vi "Configure.vi"(8 "error in (no error)":errorcluster, 11 "Autofocus in":refnum<class "Autofocus.lvclass">) -> (0 "error out":errorcluster, 2 "cancelled?":bool, 3 "Autofocus out":refnum<class "Autofocus.lvclass">)   [LabVIEW 2012, in "Autofocus.lvclass"]
doc: "The configure method configures the details for the RabbitMQ connection, the observers and the mapping script.\n\nIn the derived class, make a call to the parent for setting these parameters."
uses:
  Autofocus.lvclass
  number of subregions.ctl
  <vilib>/Utility/miscctls.llb/LVPointTypeDef.ctl
  Autofocus.lvclass/Autofocus.ctl
  <vilib>/Distrio/Murmex/Murmex/Murmex.lvclass
panel:
  in  "button::ok":bool
  in  "button::configure murmex":bool
  in  "button::cancel":bool
  in  "Tab Control":enum32{"Component IDs", "Search parameters"}(tab)
  in  "AOTF component name":string
  in  "Camera component name":string
  in  "Stages component name":string
  in  "Epsilon (HC)":dbl
  in  "Epsilon (GS)":dbl
  in  "Number of subregions":T1 items=["4"=4, "5"=5]
  # "RabbitMQ parameters"
  # "Window position"
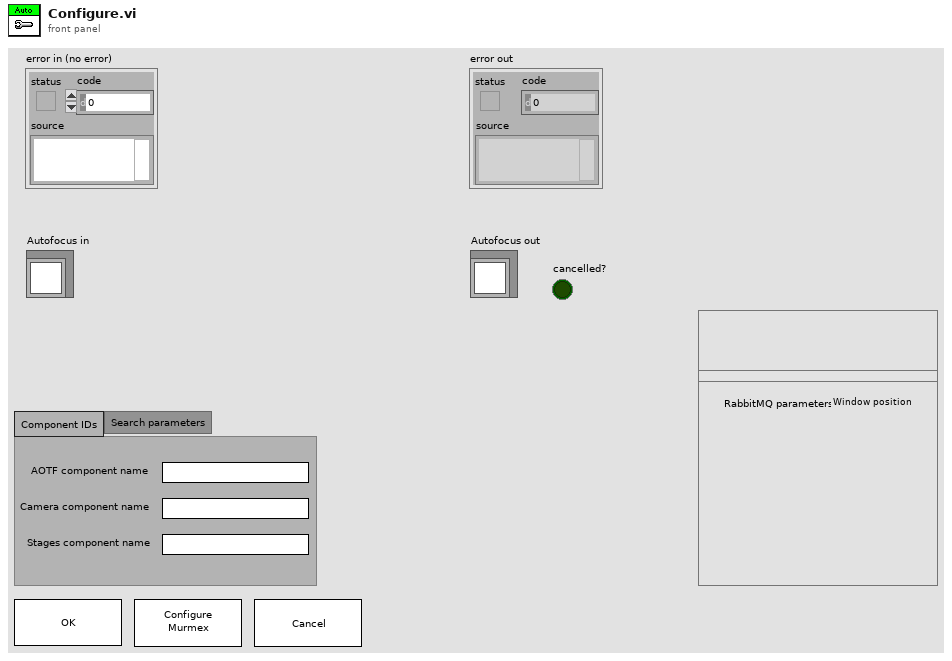
[diagram p1: front panel]
types:
  T1 = typedef "Autofocus.lvclass/number of subregions.ctl" = i32
  T2 = typedef "LVPointTypeDef.ctl" = cluster{"Horizontal":i16, "Vertical":i16}
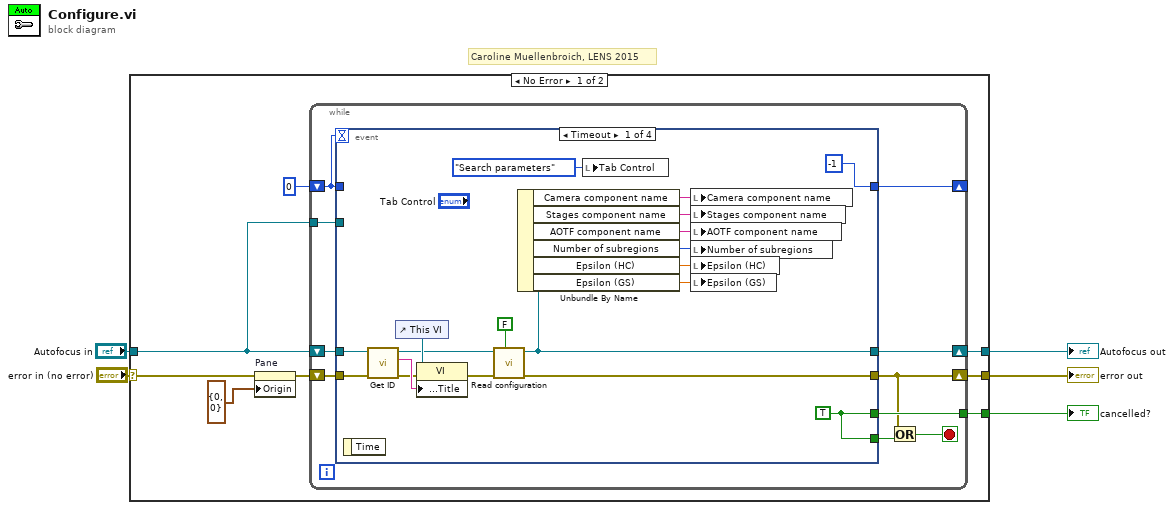
[diagram p0: block diagram]
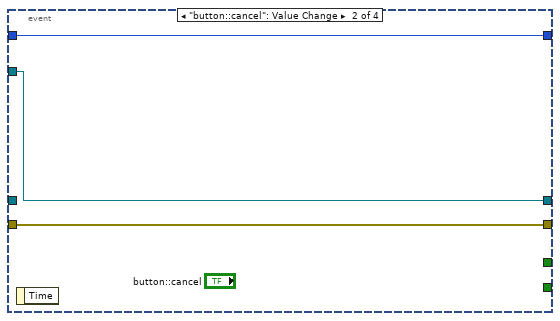
[diagram p2: hidden frame]
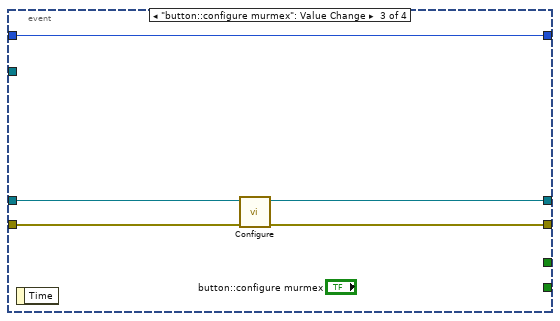
[diagram p3: hidden frame]
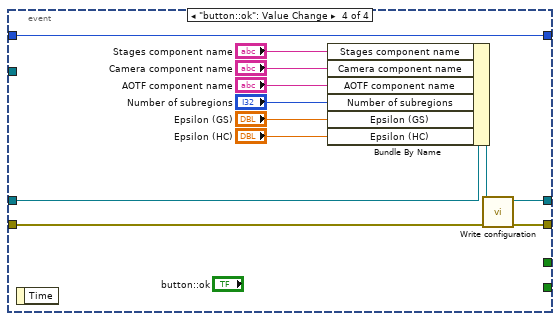
[diagram p4: hidden frame]
diagram:
  # "Caroline Muellenbroich, LENS 2015"
  n1 = case shown="No Error" "error in (no error)" {
    selector: "error in (no error)" -> [w12 w64]
    tunnel: "Autofocus in" -> [w10 w63]
    tunnel: [w8 w64] -> w3
    tunnel: [w7 w63] -> w2
    tunnel: [w6 _] -> w1
    frame No Error {
      n2 = property on="Pane" class="Pane"(error in=w12, "Origin"=T2 {"Horizontal"=0, "Vertical"=0}) -> (error out=w11:errorcluster)  [unwired: 1 in, 1 out]
      n3 = while {
        shift-right: [w18] -> w7
        shift-left: w10 -> [w20]
        shift-right: [w15] -> w8
        shift-left: w11 -> [w21]
        tunnel: w10 -> [w23]
        shift-right: [w19] -> _
        shift-left: 0 -> [w22]
        tunnel: [w17] -> w6
        stop <- w16 stop-if-true
        n4 = event shown="[0] Timeout" {
          selector: _ -> [_ _ _ _]
          dyn-events: _ -> [_ _ _ _]
          timeout: w22 -> [_ _ _ _]
          tunnel: w23 -> [_ w43 _ _]
          tunnel: w22 -> [_ w44 w46 w57]
          tunnel: w21 -> [w40 w45 w50 w60]
          tunnel: w20 -> [w39 _ w48 w59]
          tunnel: [-1 w44 w46 w57] -> w19
          tunnel: [w33 w43 w47 w61] -> w18
          tunnel: [w32 w45 w49 w62] -> w15
          tunnel: [w31 _ _ _] -> w17
          tunnel: [w31 _ _ _] -> w14
          event Timeout {
            w31 = TRUE ("force loading?")
            n5 = event-data() -> ()  [unwired: 1 in, 1 out]
            n6 = call <vilib>:"Get ID.vi"("error in (no error)"=w40, "Murmex in"=w39) -> ("error out"=w41:errorcluster, "component id"=w42:string, "Murmex out"=w36:refnum<class "Autofocus.lvclass">)  [unwired: 7 in]
            n7 = control-ref of="This VI"() -> (w38:refnum<vi>)
            n8 = property class="VI"(reference=w38, error in=w41, "Front Panel.Title"=w42) -> (error out=w37:errorcluster)  [unwired: 1 out]
            n9 = call-dynamic "Read configuration.vi"("force loading?"=FALSE, "error in (no error)"=w37, "Autofocus in"=w36) -> ("error out"=w32:errorcluster, "Autofocus out"=w33:refnum<class "Autofocus.lvclass">)  [unwired: 7 in]
            n10 = Unbundle By Name(w33) -> ("Camera component name"=w29:string, "Stages component name"=w28:string, "AOTF component name"=w27:string, "Number of subregions"=w26:T1, "Epsilon (HC)"=w25:dbl, "Epsilon (GS)"=w24:dbl)
            n11 = local write "Tab Control"(enum32{"Component IDs", "Search parameters"}."Search parameters" ("Tab Control")) -> ()
            n12 = local write "Camera component name"(w29) -> ()
            n13 = local write "Stages component name"(w28) -> ()
            n14 = local write "AOTF component name"(w27) -> ()
            n15 = local write "Number of subregions"(w26) -> ()
            n16 = local write "Epsilon (HC)"(w25) -> ()
            n17 = local write "Epsilon (GS)"(w24) -> ()
          }
          event "button::cancel": Value Change {
            n18 = event-data() -> ()  [unwired: 1 in, 1 out]
          }
          event "button::configure murmex": Value Change {
            n19 = event-data() -> ()  [unwired: 1 in, 1 out]
            n20 = call-parent "Configure.vi"("error in (no error)"=w50, "Murmex in"=w48) -> ("error out"=w49:errorcluster, "Murmex out"=w47:refnum<class "Autofocus.lvclass">)  [unwired: 7 in, 1 out]
          }
          event "button::ok": Value Change {
            n21 = event-data() -> ()  [unwired: 1 in, 1 out]
            n22 = Bundle By Name(cluster=w59, "Stages component name"="Stages component name", "Camera component name"="Camera component name", "AOTF component name"="AOTF component name", "Number of subregions"="Number of subregions", "Epsilon (GS)"="Epsilon (GS)", "Epsilon (HC)"="Epsilon (HC)") -> (w58:refnum<class "Autofocus.lvclass">)
            n23 = call-dynamic "Write configuration.vi"("error in (no error)"=w60, "Autofocus in"=w58) -> ("error out"=w62:errorcluster, "Autofocus out"=w61:refnum<class "Autofocus.lvclass">)  [unwired: 8 in]
          }
        }
        n24 = Or(x=w15, y=w14) -> (x .or. y?=w16:bool)
      }
    }
    frame Error {
    }
  }
  "error out" <- w3
  "Autofocus out" <- w2
  "cancelled?" <- w1
